vi "Sync Tasks-Trig Skew Correction.vi"(4 "Reference Clock Rate":dbl=100000000.0, 6 "Reference Clock Source":tag="PXIe_Clk100", 8 "error in":errorcluster, 11 "Task(s) in":refnum<k21>[](array[refnum])) -> (0 "error out":errorcluster, 3 "Task(s) out":refnum<k21>[](array[refnum]))   [LabVIEW 2022 SP3]
doc: "This subVI synchronizes multiple tasks together using Reference Clock Synchronization and Trigger Skew Correction. With Reference Clock Synchronization providing tight synchronization of each device's timing source, the two tasks are very well synchronized. Trigger Skew Correction sacrifices latency, generally up to 2 ticks of PXIe_Sync100, for determinism while sharing triggers. The first task in the array of tasks is assumed to be the master."
uses:
  <resource>/objmgr/daqmx.rc
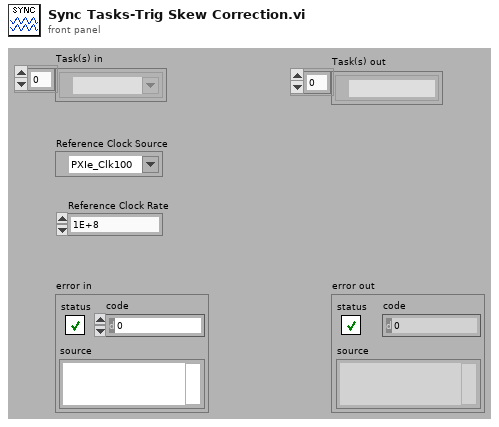
[diagram p1: front panel]
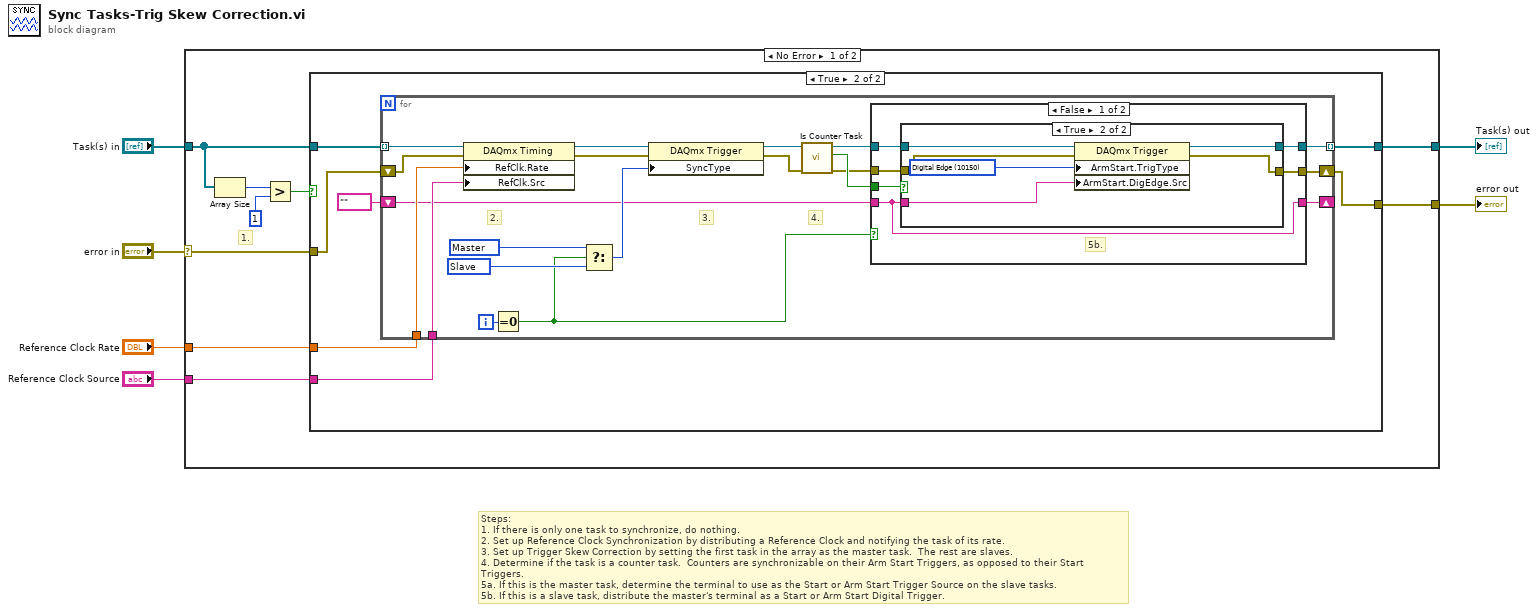
[diagram p0: block diagram]
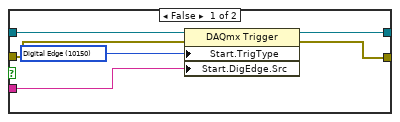
[diagram p3: hidden frame]
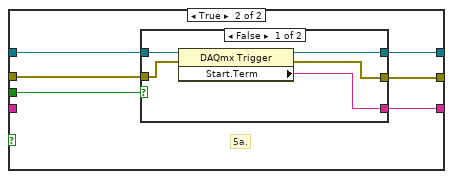
[diagram p4: hidden frame]
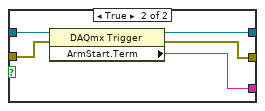
[diagram p5: hidden frame]
diagram:
  # "Steps:\n1. If there is only one task to synchronize, do nothing.\n2. Set up Reference Clock Synchronization by distributing a Reference Clock and notifying the task of its rate.\n3. Set up Trigger Skew Correction by setting the first task in the array as the master task.  The rest are slaves.\n4. Determine if the task is a counter task.  Counters are synchronizable on their Arm Start Triggers, as opposed to their Start Triggers.\n5a. If this is the master task, determine the terminal to use as the Start or Arm Start Trigger Source on the slave tasks.\n5b. If this is a slave task, distribute the master's terminal as a Start or Arm Start Digital Trigger."
  n1 = case shown="No Error" "error in" {
    selector: "error in" -> [w9 w80]
    tunnel: [w10 w80] -> w5
    tunnel: [w11 w79] -> w4
    tunnel: "Task(s) in" -> [w12 w79]
    tunnel: "Reference Clock Source" -> [w7 _]
    tunnel: "Reference Clock Rate" -> [w8 _]
    frame No Error {
      # "1."
      n2 = Array Size(array=w12) -> (size(s)=w15:i32)
      n3 = Greater?(x=w15, y=1) -> (0:w13:bool)
      n4 = case shown="True" w13 {
        tunnel: w12 -> [w17 w22]
        tunnel: [w17 w20] -> w11
        tunnel: [w16 w19] -> w10
        tunnel: w9 -> [w16 w21]
        tunnel: w8 -> [_ w23]
        tunnel: w7 -> [_ w24]
        frame False {
        }
        frame True {
          n5 = for {
            shift-right: [w28] -> w19
            shift-left: w21 -> [w35]
            tunnel: w24 -> [w42]
            tunnel: w23 -> [w41]
            tunnel: w22 -> [w36] mode=indexing
            tunnel: [w27] -> w20 mode=indexing
            shift-right: [w26] -> _
            shift-left: tag "" ("ArmStart.Term") -> [w25]
            i -> [w40]
            w38 = 15888 items=["None"=10230, "Master"=15888, "Slave"=15889] ("SyncType")
            w39 = 15889 items=["None"=10230, "Master"=15888, "Slave"=15889] ("SyncType")
            # "4."
            # "3."
            # "2."
            n6 = property class="DAQmx Timing"(reference=w36, error in=w35, "RefClk.Rate"=w41, "RefClk.Src"=w42) -> (reference out=w43:refnum<k21>, error out=w44:errorcluster)
            n7 = Equal To 0?(x=w40) -> (x = 0?=w32:bool)
            n8 = Select(t=w38, s=w32, f=w39) -> (s? t:f=w37:i32)
            n9 = property class="DAQmx Trigger"(reference=w43, error in=w44, "SyncType"=w37) -> (reference out=w34:refnum<k21>, error out=w33:errorcluster)
            n10 = call "Is Counter Task.vi"("error in"=w33, "Task"=w34) -> ("error out"=w30:errorcluster, "Is Counter Task"=w31:bool, "Task"=w29:refnum<k21>)  [unwired: 7 in]
            n11 = case shown="False" w32 {
              tunnel: w31 -> [w50 w68]
              tunnel: w30 -> [w46 w67]
              tunnel: w29 -> [w49 w66]
              tunnel: [w47 w65] -> w28
              tunnel: [w48 w64] -> w27
              tunnel: [w45 w63] -> w26
              tunnel: w25 -> [w45 _]
              frame False {
                # "5b."
                n12 = case shown="True" w50 {
                  tunnel: w49 -> [w56 w62]
                  tunnel: [w55 w61] -> w48
                  tunnel: [w54 w60] -> w47
                  tunnel: w46 -> [w53 w59]
                  tunnel: w45 -> [w52 w58]
                  frame False {
                    w51 = 10150 items=["Analog Edge"=10099, "Digital Edge"=10150, "Digital Pattern"=10398, "Analog Window"=10103, "None"=10230] ("Start.TrigType")
                    n13 = property class="DAQmx Trigger"(reference=w56, error in=w53, "Start.TrigType"=w51, "Start.DigEdge.Src"=w52) -> (reference out=w55:refnum<k21>, error out=w54:errorcluster)
                  }
                  frame True {
                    w57 = 10150 items=["Digital Edge"=10150, "None"=10230] ("ArmStart.TrigType")
                    n14 = property class="DAQmx Trigger"(reference=w62, error in=w59, "ArmStart.TrigType"=w57, "ArmStart.DigEdge.Src"=w58) -> (reference out=w61:refnum<k21>, error out=w60:errorcluster)
                  }
                }
              }
              frame True {
                # "5a."
                n15 = case shown="False" w68 {
                  tunnel: [w73 w78] -> w64
                  tunnel: [w72 w77] -> w65
                  tunnel: [w71 w76] -> w63
                  tunnel: w67 -> [w69 w75]
                  tunnel: w66 -> [w70 w74]
                  frame False {
                    n16 = property class="DAQmx Trigger"(reference=w70, error in=w69) -> (reference out=w73:refnum<k21>, error out=w72:errorcluster, "Start.Term"=w71:tag)
                  }
                  frame True {
                    n17 = property class="DAQmx Trigger"(reference=w74, error in=w75) -> (reference out=w78:refnum<k21>, error out=w77:errorcluster, "ArmStart.Term"=w76:tag)
                  }
                }
              }
            }
          }
        }
      }
    }
    frame Error {
    }
  }
  "Task(s) out" <- w4
  "error out" <- w5
